vi "Pictures And Decorations.vi"(11 "Numeric":dbl) -> (3 "Numeric 2":dbl)   [LabVIEW 2024]
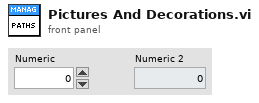
[diagram p1: front panel]
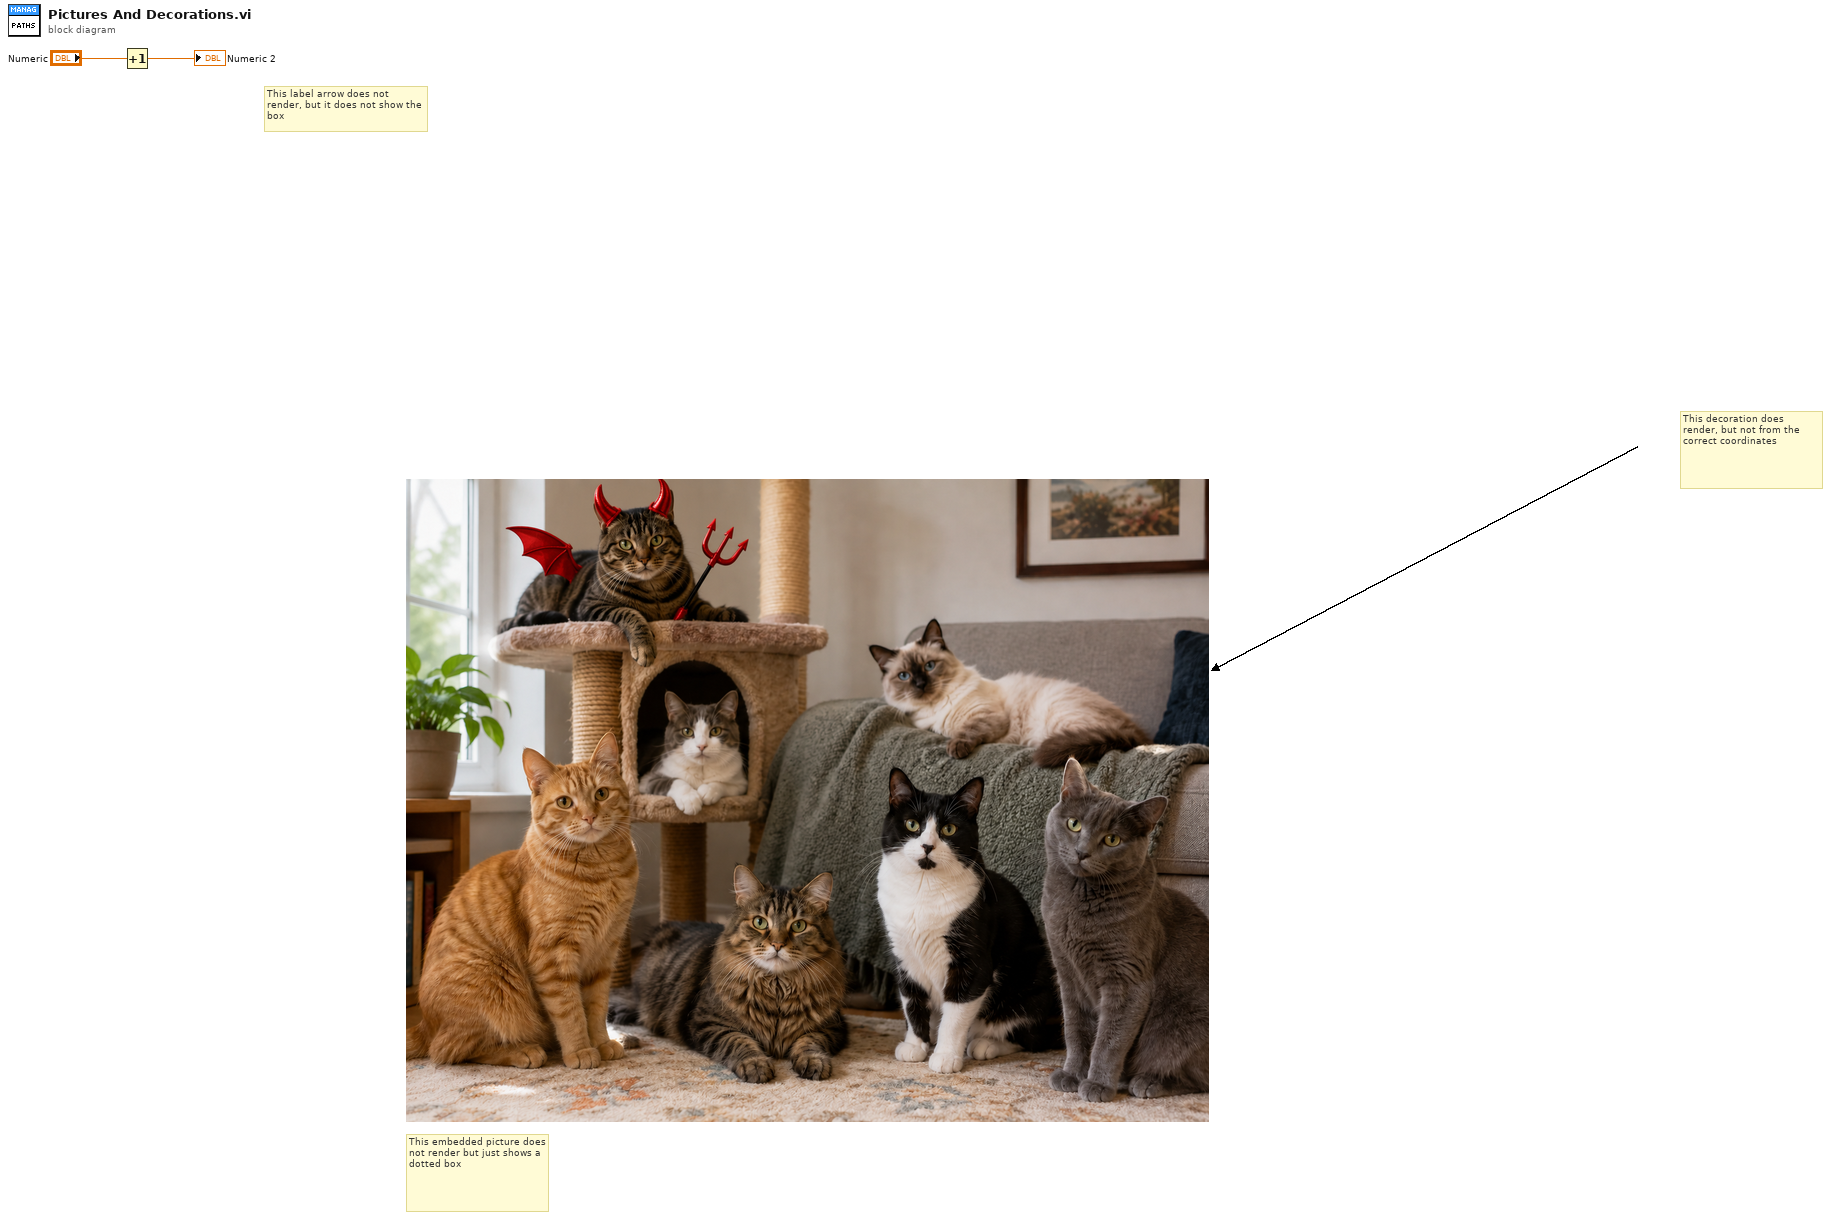
[diagram p0: block diagram]
diagram:
  # "This embedded picture does not render but just shows a dotted box"
  # "This decoration does render, but not from the correct coordinates"
  # "This label arrow does not render, but it does not show the box"
  n1 = Increment(x="Numeric") -> (x+1=→"Numeric 2":dbl)
